vi "Not a Refnum.vi"(4 "Priority Queue.lvclass":refnum<class "Priority Queue.lvclass">) -> (1 "NaN/Path/Refnum?":bool)   [LabVIEW 2020, in "Communicable State Machine.lvlib" / "Priority Queue.lvclass"]
uses:
  Priority Queue.lvclass
  Priority Queue.lvclass/Priority Queue.ctl
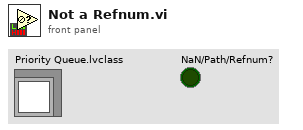
[diagram p1: front panel]
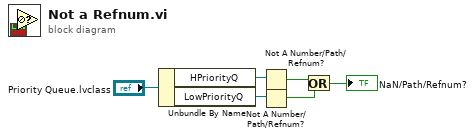
[diagram p0: block diagram]
diagram:
  n1 = Unbundle By Name("Priority Queue.lvclass") -> ("HPriorityQ"=w5:refnum<queue>, "LowPriorityQ"=w4:refnum<queue>)
  n2 = Not A Number/Path/Refnum?(number/path/refnum=w5) -> (NaN/Path/Refnum?=w3:bool)
  n3 = Not A Number/Path/Refnum?(number/path/refnum=w4) -> (NaN/Path/Refnum?=w2:bool)
  n4 = Or(x=w3, y=w2) -> (x .or. y?=→"NaN/Path/Refnum?":bool)
